vi "log.vi"(8 "error in (no error)":errorcluster, 10 "Message":string, 11 "Mission in":refnum<class "Mission.lvclass">) -> (0 "error out":errorcluster, 3 "Mission out":refnum<class "Mission.lvclass">)   [LabVIEW 2011, in "Mission.lvclass"]
doc: "Writes a log string to internal storage of the mission with an attached timestamp."
uses:
  Mission.lvclass
  Mission.lvclass/Mission.ctl
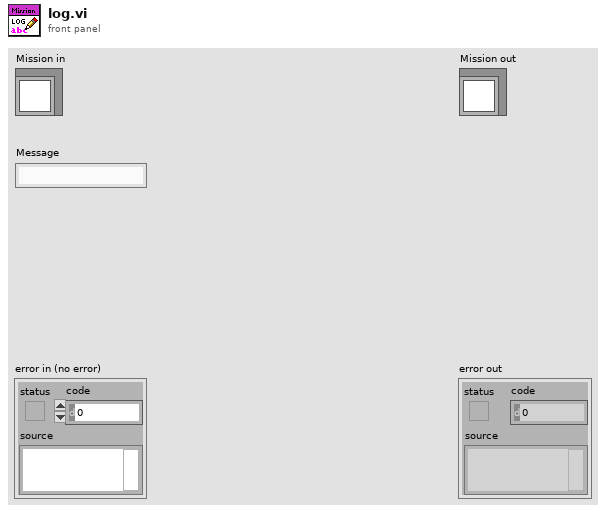
[diagram p1: front panel]
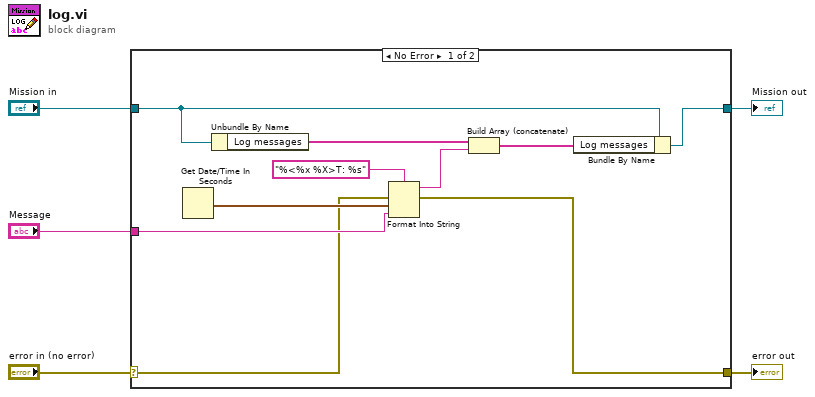
[diagram p0: block diagram]
diagram:
  n1 = case shown="No Error" "error in (no error)" {
    selector: "error in (no error)" -> [w7 w17]
    tunnel: [w6 w17] -> w4
    tunnel: [w14 w16] -> w2
    tunnel: "Mission in" -> [w15 w16]
    tunnel: "Message" -> [w9 _]
    frame No Error {
      n2 = Get Date/Time In Seconds() -> (seconds since 1Jan1904=w10:timestamp)
      n3 = Unbundle By Name(w15) -> ("Log messages"=w13:string[])
      n4 = Format Into String(format string="%<%x %X>T: %s", error in=w7, w10, w9) -> (resulting string=w8:string, error out=w6:errorcluster)  [unwired: 1 in]
      n5 = Build Array (concatenate)(w13, w8) -> (w12:string[])
      n6 = Bundle By Name(cluster=w15, "Log messages"=w12) -> (w14:refnum<class "Mission.lvclass">)
    }
    frame Error {
    }
  }
  "error out" <- w4
  "Mission out" <- w2
